vi "VDH-storeCalibration.vi"(8 "error in (no error)":errorcluster, 9 "comment":string="Comment", 10 "Calibration File Path":path, 11 "VDH-VNA_data_handler in":refnum<class "VDH-VNA_data_handler.lvclass">) -> (0 "error out":errorcluster, 3 "VDH-VNA_data_handler out":refnum<class "VDH-VNA_data_handler.lvclass">)   [LabVIEW 2020, in "VDH-VNA_data_handler.lvlib" / "VDH-VNA_data_handler.lvclass"]
uses:
  VDH-VNA_data_handler.lvclass
  VDH-SOLT_calib_save_format.ctl
  VDH-SOLT_calib_Status.ctl
  VDH-Calibration_enum.ctl
  VDH-VNA_data_handler.lvclass/VDH-VNA_data_handler.ctl
  <vilib>/Utility/config.llb/NI_LVConfig.lvlib
  common/features/CF-common_features.lvlib
  <userlib>/_OpenG.lib/variantconfig/variantconfig.llb/openg_variant_configuration_file.lvlib
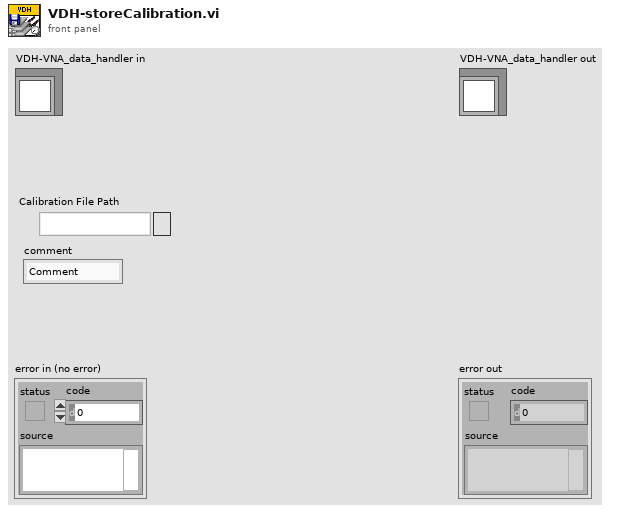
[diagram p1: front panel]
types:
  T1 = typedef "VDH-VNA_data_handler.lvlib/VDH-VNA_data_handler.lvclass/VDH-Calibration_enum.ctl" = enum16{"Non", "Short", "Open", "Load", "Through", "Permativity"}
  T2 = typedef "VDH-VNA_data_handler.lvlib/VDH-VNA_data_handler.lvclass/VDH-SOLT_calib_save_format.ctl" = cluster{"comment":string, "Calib Status":T3, "Frequency":u64[], "Short":cdb[], "Open":cdb[], "Load":cdb[], "Through":cdb[]}
  T3 = typedef "VDH-VNA_data_handler.lvlib/VDH-VNA_data_handler.lvclass/VDH-SOLT_calib_Status.ctl" = cluster{"Short":bool, "Open":bool, "Load":bool, "Through":bool}
  T4 = typedef "NI_LVConfig.lvlib/Config Data RefNum.ctl" = refnum<k1>
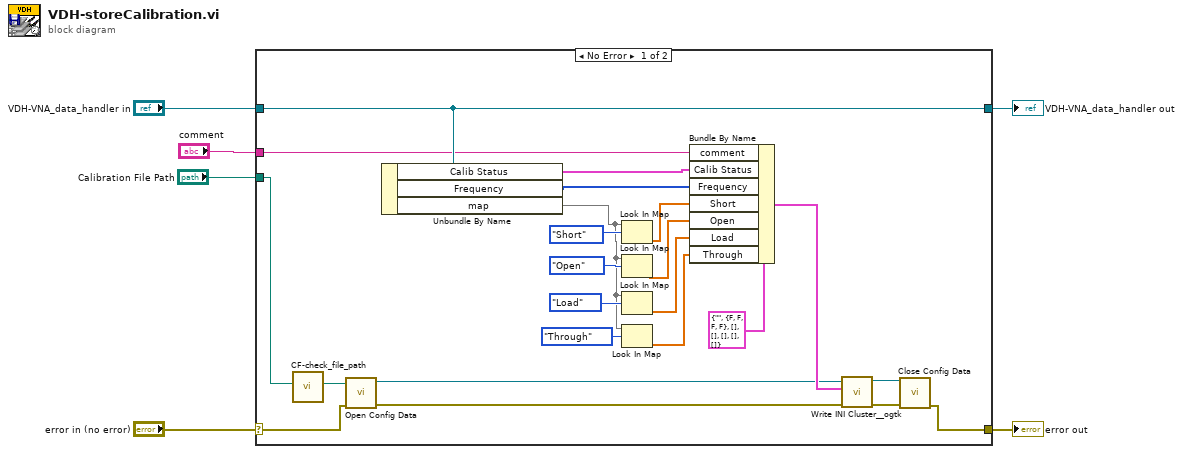
[diagram p0: block diagram]
diagram:
  n1 = case shown="No Error" "error in (no error)" {
    selector: "error in (no error)" -> [w8 w31]
    tunnel: [w9 w31] -> w5
    tunnel: [w29 w30] -> w3
    tunnel: "VDH-VNA_data_handler in" -> [w29 w30]
    tunnel: "Calibration File Path" -> [w16 _]
    tunnel: "comment" -> [w7 _]
    frame No Error {
      n2 = call "CF-check_file_path.vi"("File Path"=w16) -> ("File Path out"=w15:path)  [unwired: 10 in]
      n3 = call <vilib>:"Open Config Data.vi"("error in (no error)"=w8, "configuration file path"=w15) -> ("error out"=w13:errorcluster, "refnum"=w12:T4)  [unwired: 7 in, 1 out]
      n4 = Unbundle By Name(w29) -> ("Calib Status"=w27:T3, "Frequency"=w26:u64[], "map"=w22:map{T1, cdb[]})
      n5 = Look In Map(map=w22, key=VDH-Calibration_enum."Short" ("SOLT")) -> (value=w20:cdb[])  [unwired: 1 in, 1 out]
      n6 = Look In Map(map=w22, key=VDH-Calibration_enum."Open" ("SOLT")) -> (value=w19:cdb[])  [unwired: 1 in, 1 out]
      n7 = Look In Map(map=w22, key=VDH-Calibration_enum."Load" ("SOLT")) -> (value=w18:cdb[])  [unwired: 1 in, 1 out]
      n8 = Look In Map(map=w22, key=VDH-Calibration_enum."Through") -> (value=w17:cdb[])  [unwired: 1 in, 1 out]
      n9 = Bundle By Name(cluster=T2 {"comment"="", "Calib Status"={"Short"=FALSE, "Open"=FALSE, "Load"=FALSE, "Through"=FALSE}, "Frequency"=[], "Short"=[], "Open"=[], "Load"=[], "Through"=[]} ("SOLT save format"), "comment"=w7, "Calib Status"=w27, "Frequency"=w26, "Short"=w20, "Open"=w19, "Load"=w18, "Through"=w17) -> (w14:T2)
      n10 = call <userlib>:"Write INI Cluster__ogtk.vi"("error in (no error)"=w13, "INI Fomatted Cluster"=w14, "refnum"=w12) -> ("error out"=w10:errorcluster, "dup refnum"=w11:T4)  [unwired: 7 in]
      n11 = call <vilib>:"Close Config Data.vi"("error in (no error)"=w10, "refnum"=w11) -> ("error out"=w9:errorcluster)  [unwired: 8 in, 1 out]
    }
    frame Error {
    }
  }
  "error out" <- w5
  "VDH-VNA_data_handler out" <- w3
